vi "CNR compute bisquare weights.vi"(7 "number of parameters":i32, 8 "error in (no error)":errorcluster, 9 "weight":dbl[](array[numeric]), 10 "J":T1, 11 "raw residuals":dbl[](array[numeric])) -> (0 "error out":errorcluster, 1 "weights":dbl[](array[numeric]))   [LabVIEW 2020, in "NI_Gmath.lvlib"]
uses:
  <vilib>/gmath/NI_Gmath.lvlib
  <vilib>/Analysis/Matrix/Datatypes/RealMatrix.ctl
  <vilib>/Analysis/Matrix/NI_Matrix.lvlib
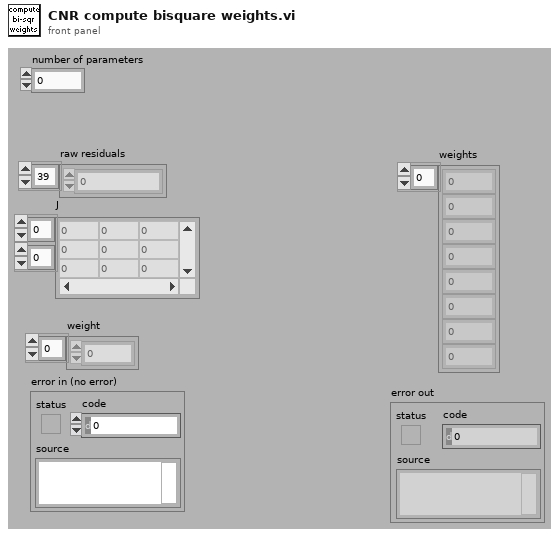
[diagram p1: front panel]
types:
  T1 = typedef "NI_Matrix.lvlib/RealMatrix.ctl" = dbl[][]
  T2 = enum16{"arithmetic", "geometric", "harmonic", "trimmed", "median"}
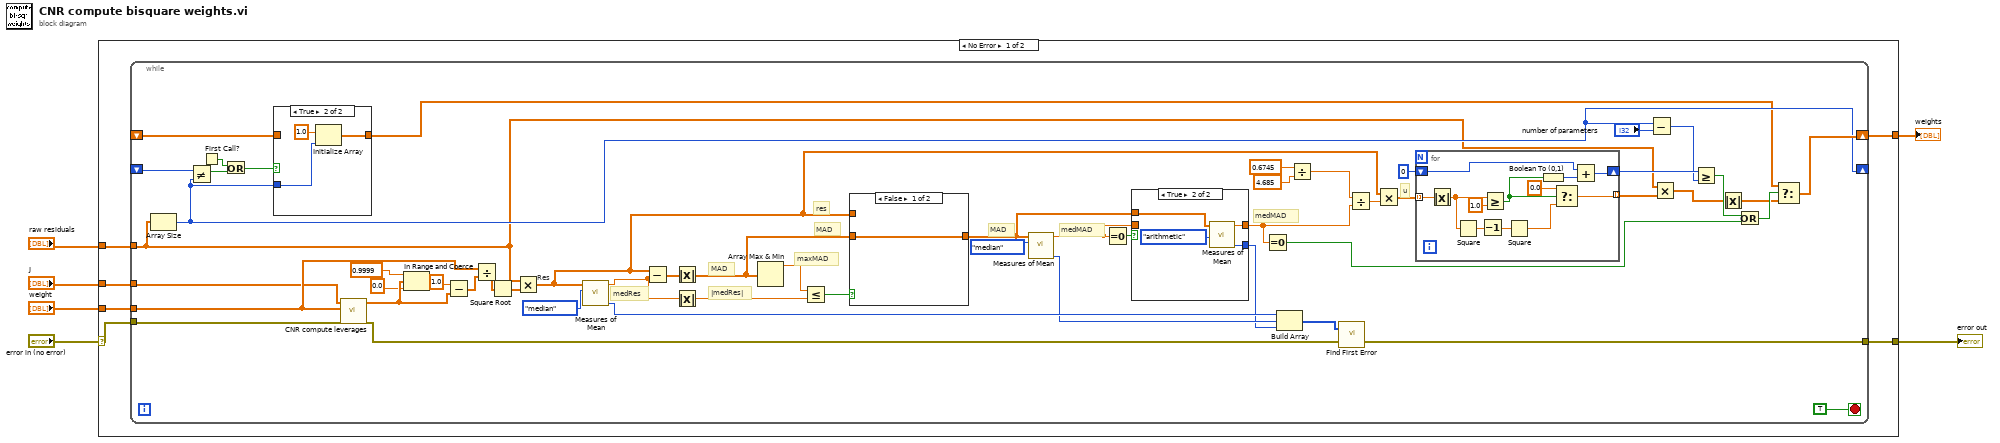
[diagram p0: block diagram]
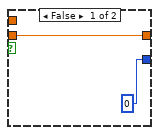
[diagram p3: hidden frame]
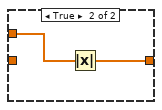
[diagram p4: hidden frame]
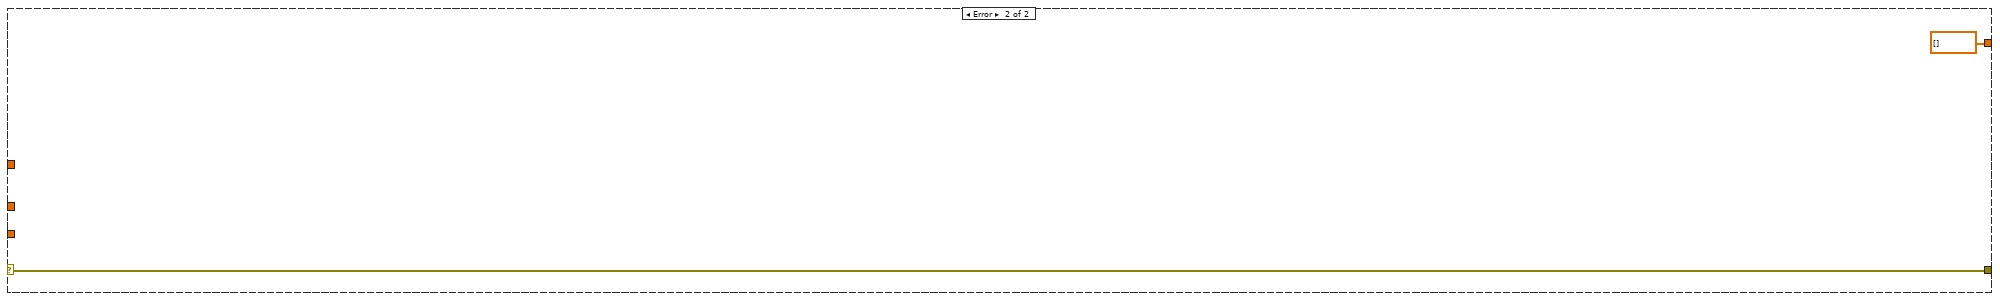
[diagram p5: hidden frame]
diagram:
  n1 = case shown="No Error" "error in (no error)" {
    selector: "error in (no error)" -> [w11 w93]
    tunnel: [w12 dbl[] []] -> w6
    tunnel: [w10 w93] -> w4
    tunnel: "weight" -> [w9 _]
    tunnel: "J" -> [w8 _]
    tunnel: "raw residuals" -> [w7 _]
    frame No Error {
      n2 = while {
        shift-right: [w42] -> w12
        shift-left: _ -> [w36]
        shift-right: [w37] -> _
        shift-left: _ -> [w41]
        tunnel: w11 -> [w18]
        tunnel: [w16] -> w10
        tunnel: w9 -> [w15]
        tunnel: w8 -> [w14]
        tunnel: w7 -> [w13]
        stop <- TRUE stop-if-true
        # "Res"
        # "u"
        # "medMAD"
        # "MAD"
        # "medMAD"
        # "MAD"
        # "res"
        # "|medRes|"
        # "MAD"
        # "medRes"
        # "maxMAD"
        n3 = Array Size(array=w13) -> (size(s)=w37:i32)
        n4 = Not Equal?(x=w41, y=w37) -> (x != y?=w40:bool)
        n5 = First Call?() -> (First Call?: T/F=w39:bool)
        n6 = Or(x=w39, y=w40) -> (x .or. y?=w38:bool)
        n7 = case shown="True" w38 {
          tunnel: w36 -> [w67 _]
          tunnel: w37 -> [_ w69]
          tunnel: [w67 w68] -> w35
          frame False {
          }
          frame True {
            n8 = Initialize Array(1.0 ("element"), w69) -> (w68:dbl[])
          }
        }
        n9 = call <vilib>:"CNR compute leverages.vi"("error in (no error)"=w18, "weight"=w15, "J"=w14) -> ("error out"=w17:errorcluster, "leverages"=w34:dbl[])  [unwired: 7 in]
        n10 = In Range and Coerce(upper limit=0.9999, x=w34, lower limit=0.0) -> ()  [unwired: 2 out]
        n11 = Subtract(x=1.0, y=w34) -> (x-y=w31:dbl[])
        n12 = Divide(x=w15, y=w31) -> (x/y=w30:dbl[])
        n13 = Square Root(x=w30) -> (sqrt(x)=w65:dbl[])
        n14 = Multiply(x=w13, y=w65) -> (x*y=w48:dbl[])
        n15 = call <vilib>:"Measures of Mean.vi"("type"=T2."median", "x array"=w48) -> ("error"=w22:i32, "mean value"=w62:dbl)  [unwired: 8 in]
        n16 = Subtract(x=w48, y=w62) -> (x-y=w63:dbl[])
        n17 = Absolute Value(x=w63) -> (abs(x)=w58:dbl[])
        n18 = Absolute Value(x=w62) -> (abs(x)=w60:dbl)
        n19 = Array Max & Min(array=w58) -> (max value=w61:dbl)  [unwired: 3 out]
        n20 = Less Or Equal?(x=w61, y=w60) -> (x <= y?=w59:bool)
        n21 = case shown="False" w59 {
          tunnel: w58 -> [w89 _]
          tunnel: w48 -> [_ w91]
          tunnel: [w89 w90] -> w55
          frame False {
          }
          frame True {
            n22 = Absolute Value(x=w91) -> (abs(x)=w90:dbl[])
          }
        }
        n23 = call <vilib>:"Measures of Mean.vi"("type"=T2."median", "x array"=w55) -> ("error"=w21:i32, "mean value"=w54:dbl)  [unwired: 8 in]
        n24 = Equal To 0?(x=w54) -> (x = 0?=w56:bool)
        n25 = case shown="True" w56 {
          tunnel: w55 -> [_ w87]
          tunnel: [w84 w86] -> w29
          tunnel: w54 -> [w84 _]
          tunnel: [0 ("error") w85] -> w20
          frame False {
          }
          frame True {
            n26 = call <vilib>:"Measures of Mean.vi"("type"=T2."arithmetic", "x array"=w87) -> ("error"=w85:i32, "mean value"=w86:dbl)  [unwired: 8 in]
          }
        }
        n27 = Equal To 0?(x=w29) -> (x = 0?=w28:bool)
        n28 = Build Array(w22, w21, w20) -> (w19:i32[])
        n29 = Divide(x=0.6745, y=4.685) -> (x/y=w50:dbl)
        n30 = call <vilib>:"Find First Error.vi"("error in (no error)"=w17, "error codes"=w19) -> ("error out"=w16:errorcluster)  [unwired: 2 in, 1 out]
        n31 = Divide(x=w50, y=w29) -> (x/y=w49:dbl)
        n32 = Multiply(x=w48, y=w49) -> (x*y=w53:dbl[])
        n33 = for {
          tunnel: w53 -> [w82] mode=indexing
          tunnel: [w76] -> w24 mode=indexing
          shift-right: [w74] -> w46
          shift-left: i16 0 -> [w72]
          n34 = Absolute Value(x=w82) -> (abs(x)=w80:dbl)
          n35 = Square(x=w80) -> (x^2=w79:dbl)
          n36 = Decrement(x=w79) -> (x-1=w78:dbl)
          n37 = Greater Or Equal?(x=w80, y=1.0) -> (x >= y?=w75:bool)
          n38 = Square(x=w78) -> (x^2=w71:dbl)
          n39 = Boolean To (0,1)(Boolean=w75) -> (0, 1=w73:i16)
          n40 = Select(t=0.0, s=w75, f=w71) -> (s? t:f=w76:dbl)
          n41 = Add(x=w72, y=w73) -> (x+y=w74:i16)
        }
        n42 = Subtract(x=w37, y="number of parameters") -> (x-y=w43:i32)
        n43 = Multiply(x=w13, y=w24) -> (x*y=w25:dbl[])
        n44 = Greater Or Equal?(x=w46, y=w43) -> (x >= y?=w27:bool)
        n45 = Absolute Value(x=w25) -> (abs(x)=w23:dbl[])
        n46 = Or(x=w27, y=w28) -> (x .or. y?=w26:bool)
        n47 = Select(t=w35, s=w26, f=w23) -> (s? t:f=w42:dbl[])
      }
    }
    frame Error {
    }
  }
  "weights" <- w6
  "error out" <- w4
